vi "Main Recipe.vi"() -> ()   [LabVIEW 2011]
panel:
  in  "Delay":dbl
  in  "Ramp":dbl
  in  "Time":dbl
  in  "Tab Control":enum32{"Steps", "Valves"}(tab)
  in  "Steps":i32(listbox)
  in  "Valves":T1(array[cluster])
  in  "Add Step":bool
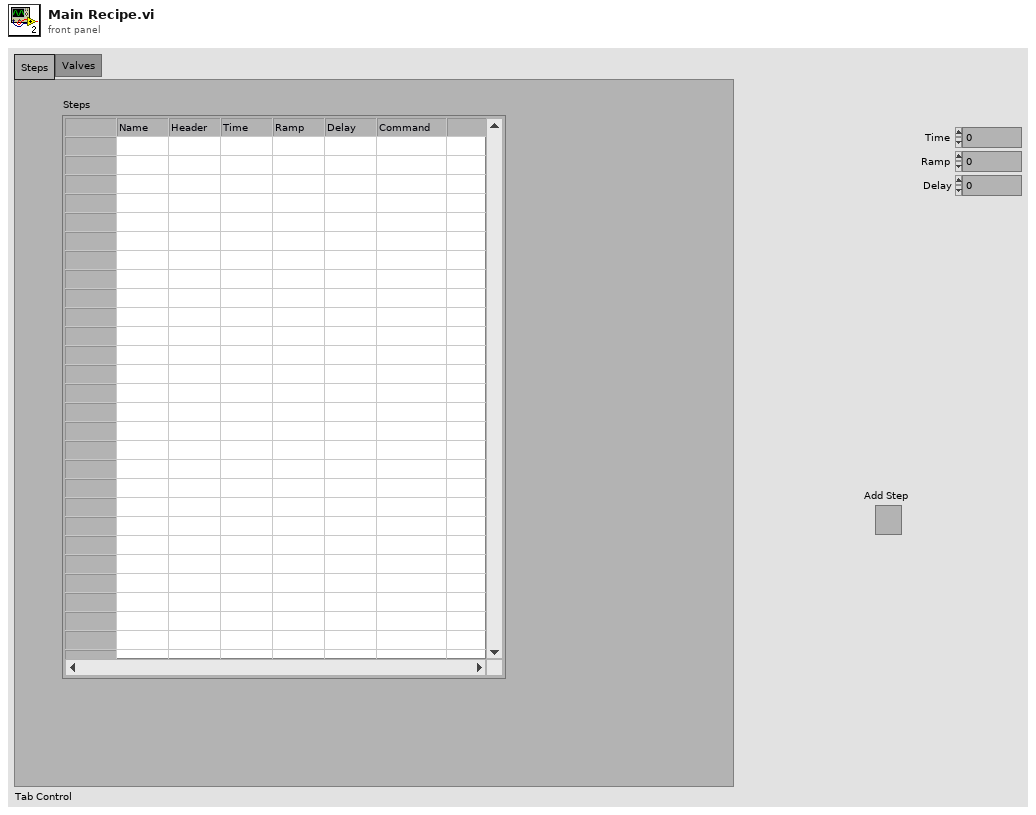
[diagram p1: front panel]
types:
  T1 = cluster{"Valve":dbl, "Enabled":bool, "Value":bool}[][]
  T2 = cluster{"Valve":i32, "Enabled":bool, "Value":bool}
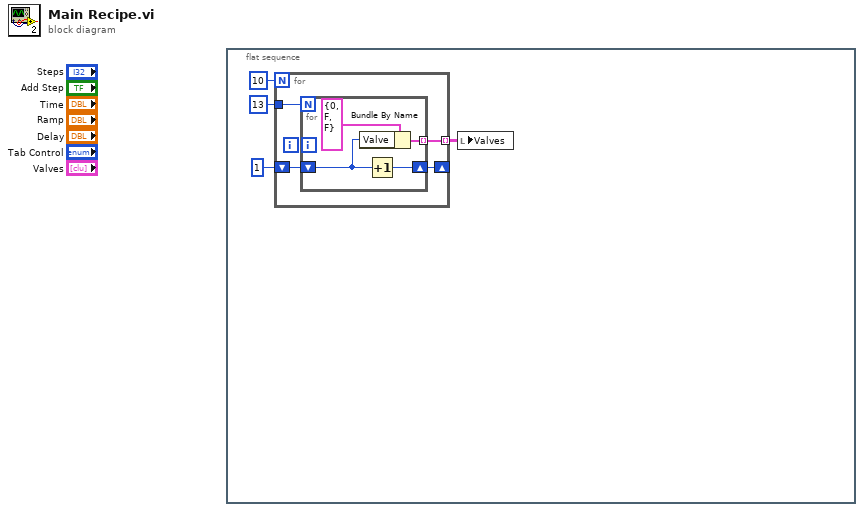
[diagram p0: block diagram]
diagram:
  n1 = flat-sequence {
    frame #0 {
      n2 = for {
        N: 10 ("dimension size") -> [_]
        tunnel: 13 ("dimension size") -> [w8]
        tunnel: [w7] -> w3 mode=indexing
        shift-right: [w5] -> _
        shift-left: 1 -> [w6]
        n3 = for {
          N: w8 -> [_]
          tunnel: [w12] -> w7 mode=indexing
          shift-right: [w10] -> w5
          shift-left: w6 -> [w9]
          n4 = Bundle By Name(cluster=T2 {"Valve"=0, "Enabled"=FALSE, "Value"=FALSE} ("Cluster"), "Valve"=w9) -> (w12:T2)
          n5 = Increment(x=w9) -> (x+1=w10:i32)
        }
      }
      n6 = local write "Valves"(w3) -> ()
    }
  }
